vi "Keithley 2002 Scan Config.vi"(1 "channel setting":u16[](array[ring]) items=["none", "Vdc", "Vac", "temp", "freq", "2-W res", "4-W res", "rjun 1", "rjun 2", "rjun 3", "rjun 4", "rjun 5", "alt"], 2 "delta meas. channel":dbl=10.0 min=1.0 max=10.0 step=1.0, 3 "ratio meas. channel":dbl=10.0 min=1.0 max=10.0 step=1.0, 4 "error in":T1, 5 "delta ref. channel":dbl=5.0 min=1.0 max=10.0 step=1.0, 6 "ratio ref. channel":dbl=5.0 min=1.0 max=10.0 step=1.0, 7 "GPIB address":string="16") -> (0 "error out":T1)   [LabVIEW 2020]
doc: "This VI is used to configure the settings for the scanning operation. Each scan channel can be set to a specific function, or even set to \"none\". The ratio and delta channels can also be changed, if either of the 2 functions will be used later.\n\nTo read the scan channels after configuring, use the Scan Read VI.\n\nNote: The array element for the Channel Setting is always 1\n less than the channel number. For example, array\n element 0 corresponds to channel number 1.\n\nThere are only 10 channels, so do not set the array past element 9."
panel:
  # "ch #"
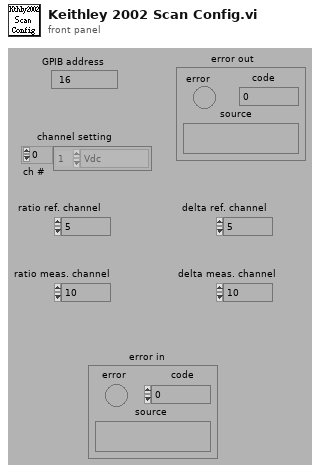
[diagram p1: front panel]
types:
  T1 = cluster{"error":bool, "code":i32, "source":string}
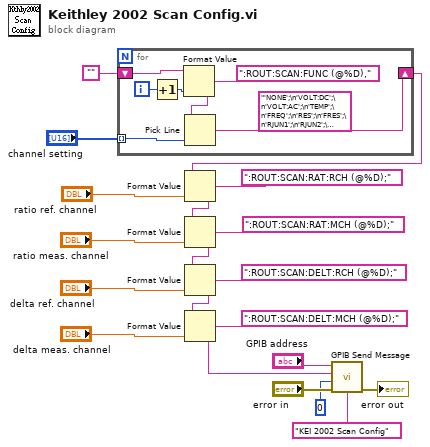
[diagram p0: block diagram]
diagram:
  n1 = for {
    tunnel: "channel setting" -> [w28] mode=indexing
    shift-right: [w21] -> w14
    shift-left: "" -> [w27]
    i -> [w26]
    n2 = Increment(x=w26) -> (x+1=w25:i32)
    n3 = Format Value(string ("")=w27, format string=":ROUT:SCAN:FUNC (@%D),", value (0)=w25) -> (output string=w23:string)
    n4 = Pick Line(string ("")=w23, multi-line string="'NONE';\n'VOLT:DC';\n'VOLT:AC';\n'TEMP';\n'FREQ';\n'RES';\n'FRES';\n'RJUN1';\n'RJUN2';\n'RJUN3';\n'RJUN4';\n'RJUN5';\n'ALT';", line index=w28) -> (output string=w21:string)
  }
  n5 = Format Value(string ("")=w14, format string=":ROUT:SCAN:RAT:RCH (@%D);", value (0)="ratio ref. channel") -> (output string=w13:string)
  n6 = Format Value(string ("")=w13, format string=":ROUT:SCAN:RAT:MCH (@%D);", value (0)="ratio meas. channel") -> (output string=w12:string)
  n7 = Format Value(string ("")=w12, format string=":ROUT:SCAN:DELT:RCH (@%D);", value (0)="delta ref. channel") -> (output string=w11:string)
  n8 = Format Value(string ("")=w11, format string=":ROUT:SCAN:DELT:MCH (@%D);", value (0)="delta meas. channel") -> (output string=w7:string)
  n9 = call "GPIB Send Message.vi"("address string"="GPIB address", "write buffer"=w7, "source"="KEI 2002 Scan Config", "write mode (set END:0)"=0, "error in"="error in") -> ("error out"=→"error out":T1)  [unwired: 2 in, 2 out]
